vi "SaveReadPrefs.vi"(3 "Task":enum16{"Read", "Save"}(ring)) -> (0 "Masters":string[](array[string]))   [LabVIEW 2012]
uses:
  <userlib>/ROS for LabVIEW Software/ROS/Code/_ROSDefinition.vi
panel:
  out "error out":errorcluster
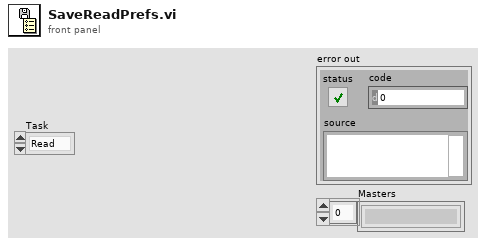
[diagram p1: front panel]
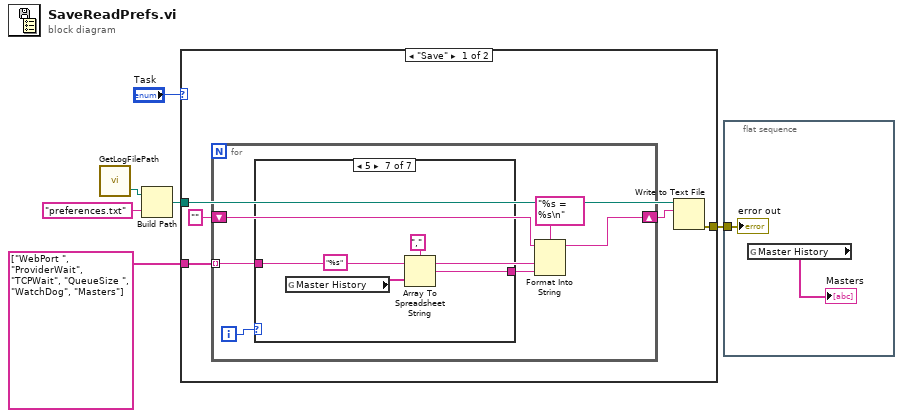
[diagram p0: block diagram]
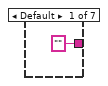
[diagram p2: hidden frame]
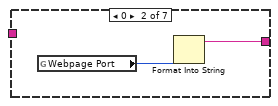
[diagram p3: hidden frame]
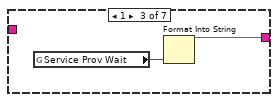
[diagram p4: hidden frame]
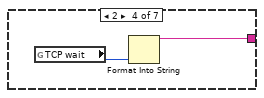
[diagram p5: hidden frame]
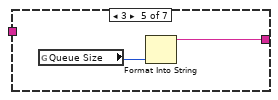
[diagram p6: hidden frame]
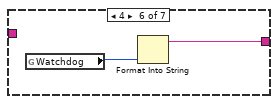
[diagram p7: hidden frame]
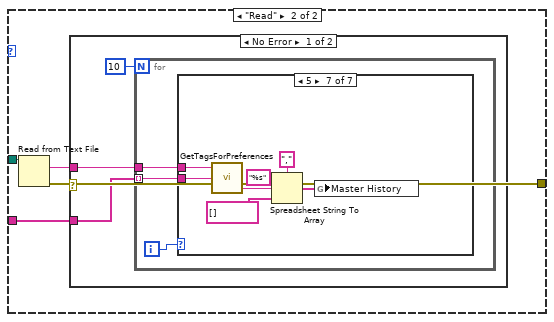
[diagram p8: hidden frame]
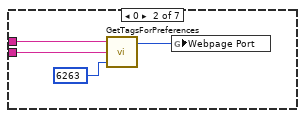
[diagram p10: hidden frame]
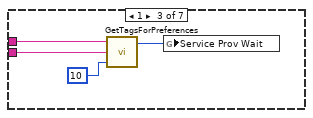
[diagram p11: hidden frame]
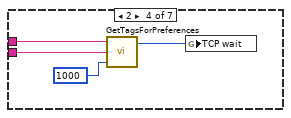
[diagram p12: hidden frame]
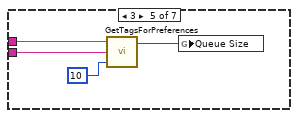
[diagram p13: hidden frame]
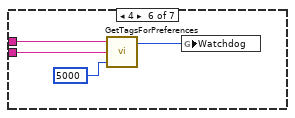
[diagram p14: hidden frame]
diagram:
  n1 = call <userlib>:"GetLogFilePath.vi"() -> ("LogFolder"=w6:path)  [unwired: 2 in, 1 out]
  n2 = Build Path(base path=w6, name or relative path="preferences.txt") -> (appended path=w4:path)
  n3 = case shown="\"Save\"" "Task" {
    tunnel: w4 -> [w9 w36]
    tunnel: string[] ["WebPort ", "ProviderWait", "TCPWait", "QueueSize ", "WatchDog", "Masters"] -> [w11 w34]
    tunnel: [w8 w33] -> w1
    frame "Save" {
      n4 = for {
        tunnel: w11 -> [w15] mode=indexing
        shift-right: [w13] -> w10
        shift-left: "" -> [w12]
        i -> [w17]
        n5 = case shown="5" w17 {
          tunnel: w15 -> [_ _ _ _ _ _ _]
          tunnel: ["" ("spreadsheet string") w19 w22 w24 w26 w28 w29] -> w14
          frame Default {
          }
          frame 0 {
            n6 = global read "_ROSDefinition.vi" "Webpage Port"() -> (w20:u16)
            n7 = Format Into String(w20) -> (resulting string=w19:string)  [unwired: 3 in, 1 out]
          }
          frame 1 {
            n8 = global read "_ROSDefinition.vi" "Service Prov Wait"() -> (w21:i32)
            n9 = Format Into String(w21) -> (resulting string=w22:string)  [unwired: 3 in, 1 out]
          }
          frame 2 {
            n10 = global read "_ROSDefinition.vi" "TCP wait"() -> (w23:i32)
            n11 = Format Into String(w23) -> (resulting string=w24:string)  [unwired: 3 in, 1 out]
          }
          frame 3 {
            n12 = global read "_ROSDefinition.vi" "Queue Size"() -> (w25:i32)
            n13 = Format Into String(w25) -> (resulting string=w26:string)  [unwired: 3 in, 1 out]
          }
          frame 4 {
            n14 = global read "_ROSDefinition.vi" "Watchdog"() -> (w27:i32)
            n15 = Format Into String(w27) -> (resulting string=w28:string)  [unwired: 3 in, 1 out]
          }
          frame 5 {
            n16 = global read "_ROSDefinition.vi" "Master History"() -> (w32:string[])
            n17 = Array To Spreadsheet String(delimiter (Tab)=",", array=w32, 3:"%s" ("format string")) -> (spreadsheet string=w29:string)
          }
        }
        n18 = Format Into String(format string="%s = %s\n", initial string=w12, w15, w14) -> (resulting string=w13:string)  [unwired: 1 in, 1 out]
      }
      n19 = Write to Text File(file (use dialog)=w9, text=w10) -> (error out=w8:errorcluster)  [unwired: 2 in, 2 out]
    }
    frame "Read" {
      n20 = Read from Text File(file (use dialog)=w36) -> (text=w35:string, error out=w33:errorcluster)  [unwired: 3 in, 2 out]
      n21 = case shown="No Error" w33 {
        tunnel: w35 -> [w38 _]
        tunnel: w34 -> [w37 _]
        frame No Error {
          n22 = for {
            N: 10 -> [_]
            tunnel: w38 -> [w41]
            tunnel: w37 -> [w40] mode=indexing
            i -> [w42]
            n23 = case shown="5" w42 {
              tunnel: w41 -> [_ w46 w50 w54 w58 w62 w69]
              tunnel: w40 -> [_ w43 w47 w51 w55 w59 w68]
              frame Default {
              }
              frame 0 {
                n24 = call <userlib>:"GetTagsForPreferences.vi"("Default"=u16 6263 ("t"), "Tag"=w43, "File"=w46) -> ("tag value"=w44:i32)  [unwired: 1 in, 1 out]
                n25 = global write "_ROSDefinition.vi" "Webpage Port"(w44) -> ()
              }
              frame 1 {
                n26 = call <userlib>:"GetTagsForPreferences.vi"("Default"=u16 10 ("t"), "Tag"=w47, "File"=w50) -> ("tag value"=w48:i32)  [unwired: 1 in, 1 out]
                n27 = global write "_ROSDefinition.vi" "Service Prov Wait"(w48) -> ()
              }
              frame 2 {
                n28 = call <userlib>:"GetTagsForPreferences.vi"("Default"=u16 1000 ("t"), "Tag"=w51, "File"=w54) -> ("tag value"=w52:i32)  [unwired: 1 in, 1 out]
                n29 = global write "_ROSDefinition.vi" "TCP wait"(w52) -> ()
              }
              frame 3 {
                n30 = call <userlib>:"GetTagsForPreferences.vi"("Default"=u16 10 ("t"), "Tag"=w55, "File"=w58) -> ("tag value"=w56:i32)  [unwired: 1 in, 1 out]
                n31 = global write "_ROSDefinition.vi" "Queue Size"(w56) -> ()
              }
              frame 4 {
                n32 = call <userlib>:"GetTagsForPreferences.vi"("Default"=u16 5000 ("t"), "Tag"=w59, "File"=w62) -> ("tag value"=w60:i32)  [unwired: 1 in, 1 out]
                n33 = global write "_ROSDefinition.vi" "Watchdog"(w60) -> ()
              }
              frame 5 {
                n34 = call <userlib>:"GetTagsForPreferences.vi"("Tag"=w68, "File"=w69) -> ("tag"=w66:string)  [unwired: 2 in, 1 out]
                n35 = Spreadsheet String To Array(delimiter (Tab)=",", format string="%s", spreadsheet string=w66, array type (2D Dbl)=string[] [] ("Master History")) -> (array=w64:string[])
                n36 = global write "_ROSDefinition.vi" "Master History"(w64) -> ()
              }
            }
          }
        }
        frame Error {
        }
      }
    }
  }
  n37 = flat-sequence {
    tunnel: w1 -> [w71]
    frame #0 {
      n38 = global read "_ROSDefinition.vi" "Master History"() -> (→"Masters":string[])
      "error out" <- w71
    }
  }
